vi "OAT Get Gap Reference.vi"   [LabVIEW 2017, in "SoundVib_RefDataProcess.lvlib"]
doc: "Computes the gap reference of the scaled signal you acquire from a DC-coupled displacement transducer channel. You can subtract the gap reference value from a signal to calculate the actual movement that the displacement transducer measures. Wire data to the <B>scaled signal [EU]</B> input to determine the polymorphic instance to use or manually select the instance."
uses:
  <vilib>/addons/Sound and Vibration/Order Analysis/Referece Data Processing/SoundVib_RefDataProcess.lvlib
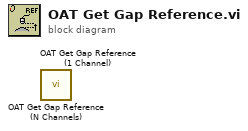
[diagram p0: block diagram]
diagram:
  n1 = call <vilib>:"OAT Get Gap Reference (N Channels).vi"() -> ()  [unwired: 14 in, 2 out]
  n2 = call <vilib>:"OAT Get Gap Reference (1 Channel).vi"() -> ()  [unwired: 14 in, 2 out]
